vi "Writing_Instrument.vi"(0 "Write String":string, 7 "Error":dbl=0.1, 11 "error in":errorcluster) -> (15 "error out":errorcluster)   [LabVIEW 2020]
doc: "This is the SubVI which is used to get in data from the input instrument and introducing an error in the input and saving it in the file"
uses:
  <vilib>/Utility/config.llb/Write Key (String).vi
  <vilib>/Utility/config.llb/NI_LVConfig.lvlib
panel:
  # "OUTPUT"
  # "INPUT"
  # "This VI gets in values introduces error and saves it in the storage file"
  # "Command: SOURce:VOLTage/CURRent:DC?"
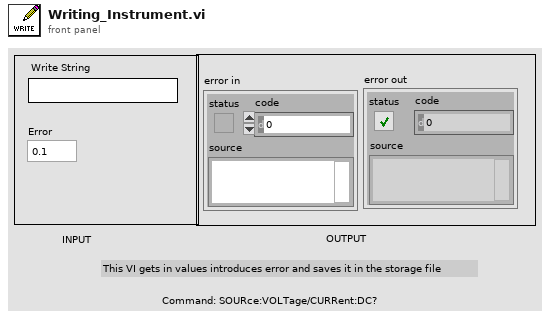
[diagram p1: front panel]
types:
  T1 = typedef "NI_LVConfig.lvlib/Config Data RefNum.ctl" = refnum<k1>
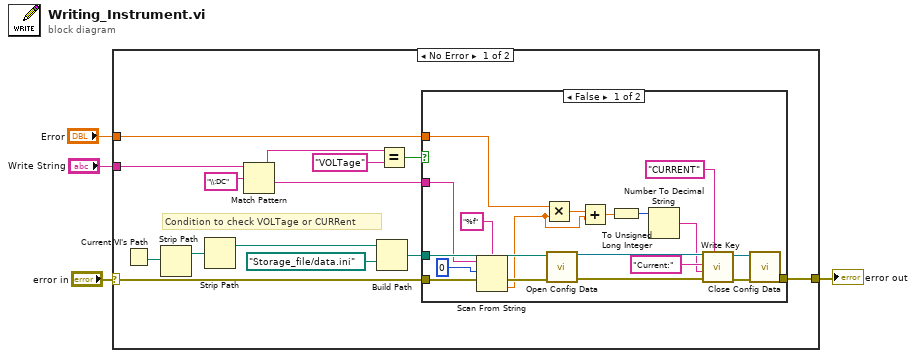
[diagram p0: block diagram]
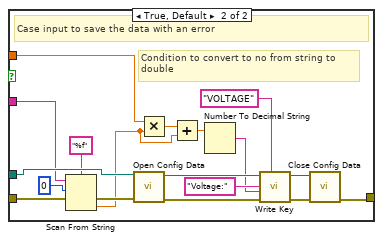
[diagram p2: hidden frame]
diagram:
  n1 = case shown="No Error" "error in" {
    selector: "error in" -> [w9 w56]
    tunnel: [w8 w56] -> w3
    tunnel: "Error" -> [w5 _]
    tunnel: "Write String" -> [w7 _]
    frame No Error {
      # "Condition to check VOLTage or CURRent"
      n2 = Current VI's Path() -> (path=w14:path)
      n3 = Strip Path(path=w14) -> (stripped path=w13:path)  [unwired: 1 out]
      n4 = Strip Path(path=w13) -> (stripped path=w12:path)  [unwired: 1 out]
      n5 = Match Pattern(string=w7, regular expression="\\:DC") -> (before substring=w17:string, after substring=w6:string)  [unwired: 1 in, 2 out]
      n6 = Build Path(base path=w12, name or relative path=path "Storage_file/data.ini") -> (appended path=w10:path)
      n7 = Equal?(x=w17, y="VOLTage") -> (x = y?=w15:bool)
      n8 = case shown="False" w15 {
        tunnel: w10 -> [w35 w53]
        tunnel: [w28 w45] -> w8
        tunnel: w9 -> [w24 w43]
        tunnel: w6 -> [w22 w41]
        tunnel: w5 -> [w21 w40]
        frame False {
          n9 = Scan From String(format string="%f", input string=w22, initial scan location=u32 0, error in=w24) -> (error out=w23:errorcluster, output 1=w19:dbl)  [unwired: 1 in, 2 out]
          n10 = Multiply(x=w21, y=w19) -> (x*y=w20:dbl)
          n11 = call <vilib>:"Open Config Data.vi"("error in (no error)"=w23, "configuration file path"=w35) -> ("error out"=w30:errorcluster, "refnum"=w31:T1)  [unwired: 7 in, 1 out]
          n12 = Add(x=w20, y=w19) -> (x+y=w26:dbl)
          n13 = To Unsigned Long Integer(number=w26) -> (unsigned 32bit integer=w25:u32)
          n14 = Number To Decimal String(number=w25) -> (decimal integer string=w29:string)  [unwired: 1 in]
          n15 = call-poly <vilib>:"Write Key.vi"("section"="CURRENT", "error in (no error)"=w30, "value"=w29, "key"="Current:" ("string"), "refnum"=w31) -> ("error out"=w36:errorcluster, "refnum out"=w37:T1)  [unwired: 4 in, 1 out]
          n16 = call <vilib>:"Close Config Data.vi"("error in (no error)"=w36, "refnum"=w37) -> ("error out"=w28:errorcluster)  [unwired: 8 in, 1 out]
        }
        frame True, Default {
          # "Condition to convert to no from string to\ndouble"
          # "Case input to save the data with an error"
          n17 = Scan From String(format string="%f", input string=w41, initial scan location=u32 0, error in=w43) -> (error out=w42:errorcluster, output 1=w38:dbl)  [unwired: 1 in, 2 out]
          n18 = call <vilib>:"Open Config Data.vi"("error in (no error)"=w42, "configuration file path"=w53) -> ("error out"=w48:errorcluster, "refnum"=w49:T1)  [unwired: 7 in, 1 out]
          n19 = Multiply(x=w40, y=w38) -> (x*y=w39:dbl)
          n20 = Add(x=w39, y=w38) -> (x+y=w52:dbl)
          n21 = Number To Decimal String(number=w52) -> (decimal integer string=w46:string)  [unwired: 1 in]
          n22 = call-poly <vilib>:"Write Key.vi"("section"="VOLTAGE", "error in (no error)"=w48, "value"=w46, "key"="Voltage:" ("string"), "refnum"=w49) -> ("error out"=w54:errorcluster, "refnum out"=w55:T1)  [unwired: 4 in, 1 out]
          n23 = call <vilib>:"Close Config Data.vi"("error in (no error)"=w54, "refnum"=w55) -> ("error out"=w45:errorcluster)  [unwired: 8 in, 1 out]
        }
      }
    }
    frame Error {
    }
  }
  "error out" <- w3
